vi "write_to_device.vi"(8 "error in (no error)":errorcluster, 10 "force writing?":bool, 11 "DAQmxWriteSignals in":refnum<class "SignalWriterMM140725DAQmx.lvclass">) -> (0 "error out":errorcluster, 1 "writing failed because finite sample task already finished?":bool, 2 "written?":bool, 3 "DAQmxWriteSignals out":refnum<class "SignalWriterMM140725DAQmx.lvclass">)   [LabVIEW 2010, in "SignalWriterMM140725DAQmx.lvclass"]
uses:
  SignalWriterMM140725DAQmx.lvclass
  <vilib>/DAQmx/write.llb/DAQmx Write (Analog 1D DBL 1Chan NSamp).vi
  <vilib>/DAQmx/write.llb/DAQmx Write (Digital 1D U8 1Chan NSamp).vi
  <vilib>/DAQmx/write.llb/DAQmx Write (Digital 1D U32 1Chan NSamp).vi
  <vilib>/DAQmx/write.llb/DAQmx Write (Analog 2D DBL NChan NSamp).vi
  <vilib>/DAQmx/write.llb/DAQmx Write (Digital 2D U8 NChan NSamp).vi
  <vilib>/DAQmx/write.llb/DAQmx Write (Digital 2D U16 NChan NSamp).vi
  <vilib>/DAQmx/write.llb/DAQmx Write (Digital 2D U32 NChan NSamp).vi
  <vilib>/daqmx/miscellaneous.llb/DAQmx Fill In Error Info.vi
  Program Files (x86)/National Instruments/LabVIEW 2010/resource/objmgr/daqmx.rc
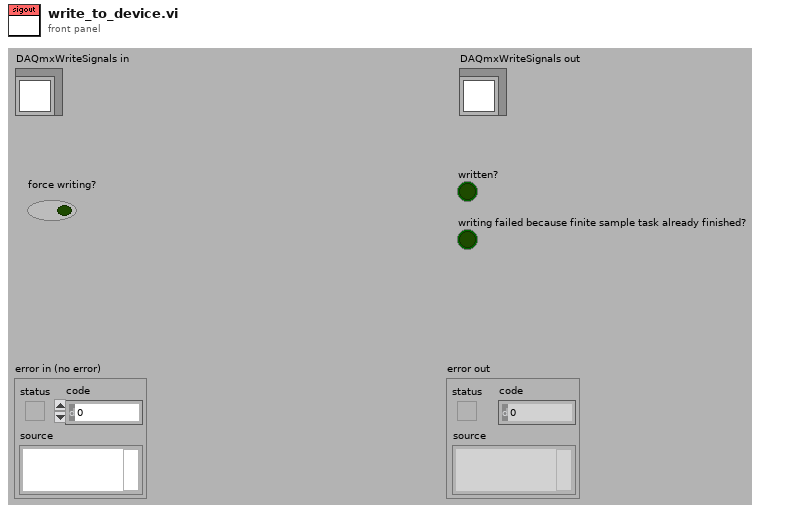
[diagram p1: front panel]
types:
  T1 = typedef "SignalWriterMM140725DAQmx.lvclass/output_type_enum.ctl" = enum16{"analog", "digital (U8)", "digital (U16)", "digital (U32)"}
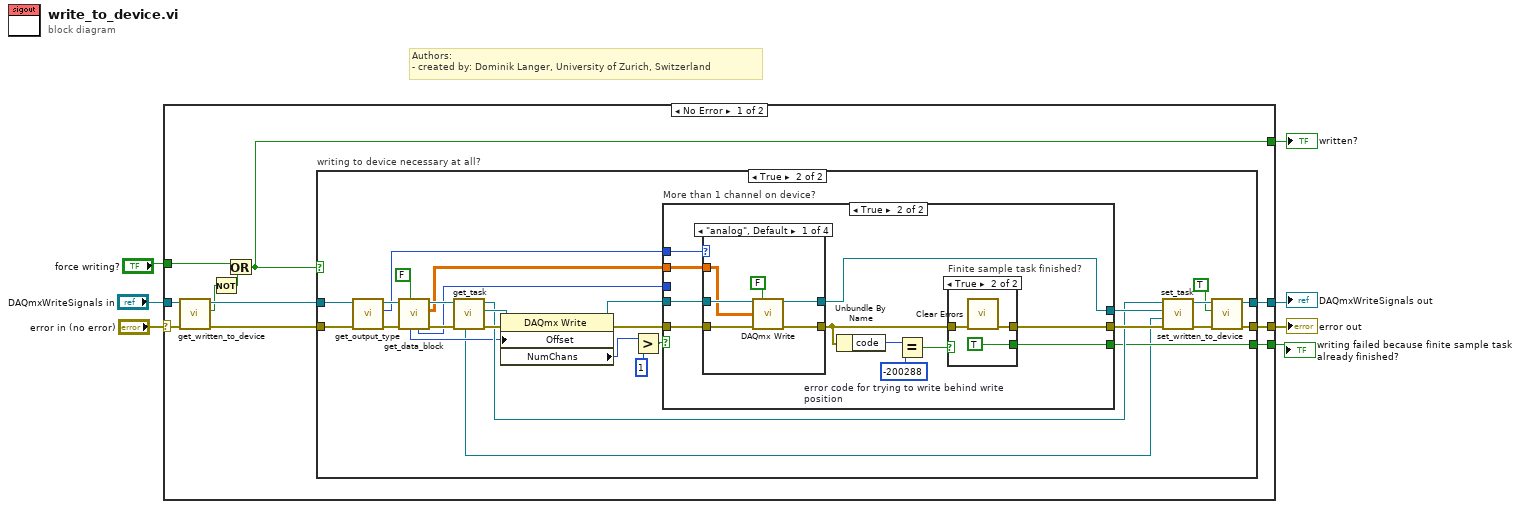
[diagram p0: block diagram]
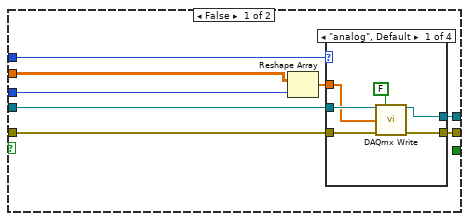
[diagram p3: hidden frame]
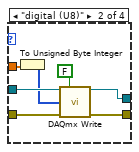
[diagram p4: hidden frame]
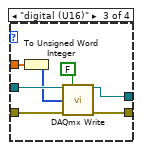
[diagram p5: hidden frame]
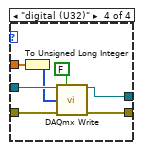
[diagram p6: hidden frame]
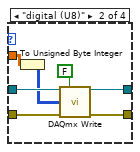
[diagram p8: hidden frame]
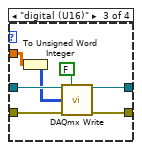
[diagram p9: hidden frame]
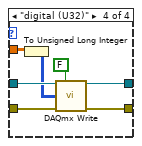
[diagram p10: hidden frame]
diagram:
  # "Authors: \n- created by: Dominik Langer, University of Zurich, Switzerland"
  n1 = case shown="No Error" "error in (no error)" {
    selector: "error in (no error)" -> [w18 w127]
    tunnel: [w10 w127] -> w5
    tunnel: [w11 w126] -> w4
    tunnel: "DAQmxWriteSignals in" -> [w16 w126]
    tunnel: [w12 _] -> w3
    tunnel: "force writing?" -> [w9 _]
    tunnel: [w8 _] -> w1
    frame No Error {
      n2 = call-dynamic "get_written_to_device.vi"("error in (no error)"=w18, "DAQmxWriteSignals in"=w16) -> ("error out"=w17:errorcluster, "written to device?"=w14:bool, "DAQmxWriteSignals out"=w15:refnum<class "SignalWriterMM140725DAQmx.lvclass">)  [unwired: 7 out]
      n3 = Not(x=w14) -> (.not. x?=w13:bool)
      n4 = Or(x=w9, y=w13) -> (x .or. y?=w12:bool)
      n5 = case "writing to device necessary at all?" shown="True" w12 {
        tunnel: [w20 w39] -> w10
        tunnel: w17 -> [w20 w31]
        tunnel: [w19 w40] -> w11
        tunnel: w15 -> [w19 w30]
        tunnel: [_ w24] -> w8
        frame False {
        }
        frame True {
          n6 = call-dynamic "get_output_type.vi"("error in (no error)"=w31, "DAQmxWriteSignals.lvclass in"=w30) -> ("error out"=w28:errorcluster, "output type"=w27:T1, "DAQmxWriteSignals.lvclass out"=w29:refnum<class "SignalWriterMM140725DAQmx.lvclass">)  [unwired: 7 out]
          n7 = call-dynamic "get_data_block.vi"("circular mode?"=FALSE, "error in (no error)"=w28, "DAQmxWriteSignals in"=w29) -> ("error out"=w33:errorcluster, "data block"=w22:dbl[][], "DAQmxWriteSignals out"=w34:refnum<class "SignalWriterMM140725DAQmx.lvclass">, "actual block size (samples)"=w32:i32, "current offset (samples)"=w35:i32)  [unwired: 4 out]
          n8 = call-dynamic "get_task.vi"("error in (no error)"=w33, "DAQmxWriteSignals in"=w34) -> ("error out"=w45:errorcluster, "writer task"=w46:refnum<k21>, "DAQmxWriteSignals out"=w37:refnum<class "SignalWriterMM140725DAQmx.lvclass">, "counter task"=w21:refnum<k21>)  [unwired: 6 out]
          n9 = property class="DAQmx Write"(reference=w46, error in=w45, "Offset"=w35) -> (reference out=w25:refnum<k21>, error out=w26:errorcluster, "NumChans"=w23:u32)
          n10 = Greater?(x=w23, y=u32 1) -> (0:w48:bool)
          n11 = case "More than 1 channel on device?" shown="True" w48 {
            tunnel: w25 -> [w54 w93]
            tunnel: w26 -> [w56 w94]
            tunnel: [w55 w90] -> w44
            tunnel: [w53 w89] -> w43
            tunnel: w22 -> [w51 w91]
            tunnel: w32 -> [w50 _]
            tunnel: w27 -> [w52 w92]
            tunnel: [_ w84] -> w24
            frame False {
              n12 = Reshape Array(w51, w50) -> (w49:dbl[])
              n13 = case shown="\"analog\", Default" w52 {
                tunnel: w56 -> [w61 w69 w75 w82]
                tunnel: [w60 w68 w74 w79] -> w55
                tunnel: w54 -> [w59 w67 w73 w81]
                tunnel: [w58 w65 w70 w80] -> w53
                tunnel: w49 -> [w57 w64 w72 w78]
                frame "analog", Default {
                  n14 = call-poly <vilib>:"DAQmx Write.vi"("task/channels in"=w59, "auto start"=FALSE, "data"=w57, "error in"=w61) -> ("task out"=w58:refnum<k21>, "error out"=w60:errorcluster)  [unwired: 10 out]
                }
                frame "digital (U8)" {
                  n15 = To Unsigned Byte Integer(number=w64) -> (unsigned 8bit integer=w63:u8[])
                  n16 = call-poly <vilib>:"DAQmx Write.vi"("task/channels in"=w67, "auto start"=FALSE, "data"=w63, "error in"=w69) -> ("task out"=w65:refnum<k21>, "error out"=w68:errorcluster)  [unwired: 10 out]
                }
                frame "digital (U16)" {
                  n17 = To Unsigned Word Integer(number=w72) -> (unsigned 16bit integer=w71:u16[])
                  n18 = call-poly <vilib>:"DAQmx Write.vi"("task/channels in"=w73, "auto start"=FALSE, "data"=w71, "error in"=w75) -> ("task out"=w70:refnum<k21>, "error out"=w74:errorcluster)  [unwired: 10 out]
                }
                frame "digital (U32)" {
                  n19 = To Unsigned Long Integer(number=w78) -> (unsigned 32bit integer=w77:u32[])
                  n20 = call-poly <vilib>:"DAQmx Write.vi"("task/channels in"=w81, "auto start"=FALSE, "data"=w77, "error in"=w82) -> ("task out"=w80:refnum<k21>, "error out"=w79:errorcluster)  [unwired: 10 out]
                }
              }
            }
            frame True {
              w86 = -200288  # error code for trying to write behind write position
              n21 = case shown="\"analog\", Default" w92 {
                tunnel: w94 -> [w103 w111 w117 w124]
                tunnel: [w102 w110 w116 w121] -> w87
                tunnel: w93 -> [w101 w109 w115 w123]
                tunnel: [w100 w107 w112 w122] -> w89
                tunnel: w91 -> [w99 w106 w114 w120]
                frame "analog", Default {
                  n22 = call-poly <vilib>:"DAQmx Write.vi"("task/channels in"=w101, "auto start"=FALSE, "data"=w99, "error in"=w103) -> ("task out"=w100:refnum<k21>, "error out"=w102:errorcluster)  [unwired: 10 out]
                }
                frame "digital (U8)" {
                  n23 = To Unsigned Byte Integer(number=w106) -> (unsigned 8bit integer=w105:u8[][])
                  n24 = call-poly <vilib>:"DAQmx Write.vi"("task/channels in"=w109, "auto start"=FALSE, "data"=w105, "error in"=w111) -> ("task out"=w107:refnum<k21>, "error out"=w110:errorcluster)  [unwired: 10 out]
                }
                frame "digital (U16)" {
                  n25 = To Unsigned Word Integer(number=w114) -> (unsigned 16bit integer=w113:u16[][])
                  n26 = call-poly <vilib>:"DAQmx Write.vi"("task/channels in"=w115, "auto start"=FALSE, "data"=w113, "error in"=w117) -> ("task out"=w112:refnum<k21>, "error out"=w116:errorcluster)  [unwired: 10 out]
                }
                frame "digital (U32)" {
                  n27 = To Unsigned Long Integer(number=w120) -> (unsigned 32bit integer=w119:u32[][])
                  n28 = call-poly <vilib>:"DAQmx Write.vi"("task/channels in"=w123, "auto start"=FALSE, "data"=w119, "error in"=w124) -> ("task out"=w122:refnum<k21>, "error out"=w121:errorcluster)  [unwired: 10 out]
                }
              }
              n29 = Unbundle By Name(w87) -> ("code"=w85:i32)
              n30 = Equal?(x=w85, y=w86) -> (x = y?=w88:bool)
              n31 = case "Finite sample task finished?" shown="True" w88 {
                tunnel: w87 -> [w95 w98]
                tunnel: [w95 w97] -> w90
                tunnel: [_ TRUE] -> w84
                frame False {
                }
                frame True {
                  n32 = call <vilib>:"Clear Errors.vi"("error in (no error)"=w98) -> ("error out"=w97:errorcluster)  [unwired: 6 out]
                }
              }
            }
          }
          n33 = call-dynamic "set_task.vi"("error in (no error)"=w44, "counter task"=w21, "output task"=w43, "DAQmxWriteSignals in"=w37) -> ("error out"=w42:errorcluster, "DAQmxWriteSignals out"=w41:refnum<class "SignalWriterMM140725DAQmx.lvclass">)  [unwired: 6 out]
          n34 = call-dynamic "set_written_to_device.vi"("error in (no error)"=w42, "written to device?"=TRUE, "DAQmxWriteSignals in"=w41) -> ("error out"=w39:errorcluster, "DAQmxWriteSignals out"=w40:refnum<class "SignalWriterMM140725DAQmx.lvclass">)  [unwired: 7 out]
        }
      }
    }
    frame Error {
    }
  }
  "error out" <- w5
  "DAQmxWriteSignals out" <- w4
  "written?" <- w3
  "writing failed because finite sample task already finished?" <- w1
